vi "Tag-FPGA-))Channel-NoOp.vi"(8 "abort (F)":bool, 10 "element in":T2, 11 "channelOp":T1) -> (0 "aborted?":bool, 2 "element out":i32, 3 "sequence":i16)   [LabVIEW 2020]
uses:
  Element.ctl
  Flex.lvlib
  ChannelOp.ctl
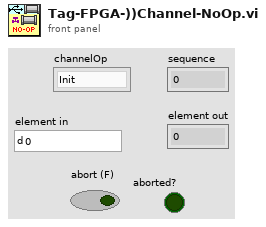
[diagram p1: front panel]
types:
  T1 = typedef "Flex.lvlib/ChannelOp.ctl" = enum16{"Init", "Close", "Probe", "New Queue"}
  T2 = typedef "Flex.lvlib/Element.ctl" = dbl
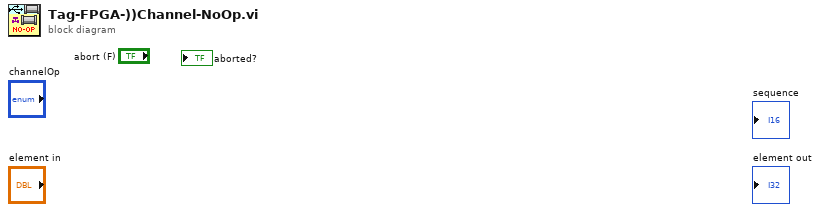
[diagram p0: block diagram]
diagram:
